vi "CD Init.vi"(8 "Error (in)":errorcluster, 11 "Device Reference":T10 format="%.0x") -> (0 "Error (out)":errorcluster, 1 "Inline Status Channels Refs":T3[](array[typedef]) format="%.0x", 2 "Card Parameters (out)":T22, 3 "RT Inline Data_Data Description_Channels":T13[](array[typedef]) {"Broadcast Frame Descriptors"."RTs"."Status Channel Ref" format="%.0x"; "Broadcast Frame Descriptors"."RTs"."Timestamp Channel Data Reference" format="%.0x"; "Broadcast Frame Descriptors"."BC"."Status Channel Refs" format="%.0x"; "Broadcast Frame Descriptors"."BC"."Words Block Data Refs"."Data Reference" format="%.0x"; "Broadcast Frame Descriptors"."BC"."Timestamp Channel Data Reference" format="%.0x"; "Frame Drescriptors"."RT"."Status Channel Ref" format="%.0x"; "Frame Drescriptors"."RT"."Words Block Data Refs"."Data Reference" format="%.0x"; "Frame Drescriptors"."RT"."Timestamp Channel Data Reference" format="%.0x"; "Frame Drescriptors"."BC"."Status Channel Refs" format="%.0x"; "Frame Drescriptors"."BC"."Words Block Data Refs"."Data Reference" format="%.0x"; "Frame Drescriptors"."BC"."Timestamp Channel Data Reference" format="%.0x"}, 6 "RT Async Data":T1 {"Map (MC Tx)"."Word Data Reference" format="%.0x"; "Map (MC Rx)"."Channel Data Reference" format="%.0x"; "Map (RT Command Channels)"."RT Command Channel Ref" format="%.0x"; "MAP (BC Acyclic Messages Trigger)"."Acyclic Message Trigger Channel Ref" format="%.0x"; "Map (Bc Command Channels)"."BC Command Channel Ref" format="%.0x"; "Map (RT to ..)"."Word Data Reference" format="%.0x"; "Map (BC to RT)"."Channel Data Reference" format="%.0x"})   [LabVIEW 2017, in "Ballard MIL-1553 Engine.lvlib"]
doc: "This VI reads all properties, creates different Maps (Tx) and initializes the Core of the board using XML file. Initialization is done here because Rx part is done Inline and Tx part asynchronously."
uses:
  Ballard MIL-1553 Engine.lvlib
  <vilib>/NI Veristand/Custom Device API/Custom Device Item Ref.ctl
  Controls/Card Parameters.ctl
  Shared/Controls and Global/Initialization Method.ctl
  Controls/RT Inline Data_Data Description_Channel.ctl
  Controls/RT Inline Frame Descriptor.ctl
  Controls/RT Inline Frame Descriptor_BC.ctl
  <vilib>/NI Veristand/Custom Device API/Data Reference.ctl
  <vilib>/NI Veristand/Custom Device API/Block Data Reference.ctl
  Controls/RT Inline Frame Descriptor_RT.ctl
  Shared/Controls and Global/RT CWD2.ctl
  Shared/Controls and Global/RT CWD1.ctl
  Shared/Controls and Global/RT messageType.ctl
  Controls/RT Inline Broadcast Frame Descriptor.ctl
  Controls/RT Async Data.ctl
  Controls/RT Async_Map BC2RT.ctl
  Controls/RT Async_Map_Type.ctl
  Controls/RT Async_Raw Values.ctl
  Controls/RT Async_Raw Values to Messages Index_Association.ctl
  Controls/RT Async_Map RT2BC.ctl
  Controls/RT Async_Map RTs Status.ctl
  Controls/RT Async_Map BC Command Channels.ctl
  Controls/RT Async_Map BC Acyclic Messages Trigger.ctl
  Controls/RT Async_Map RT Command Channels.ctl
  Controls/RT Init States.ctl
  Shared/Controls and Global/Compiled.Settings.ctl
  Shared/Controls and Global/RT Channel.ctl
  Shared/Controls and Global/RT BC.ctl
  Shared/Controls and Global/RT Message.ctl
  Shared/Controls and Global/RT Remote Terminal.ctl
  Shared/Controls and Global/RT Remote Terminal_rtMode.ctl
  Shared/Controls and Global/RT Remote Terminal_RT subAddress.ctl
  Shared/Controls and Global/RT Remote Terminal_RT direction.ctl
  Shared/Controls and Global/RT Remote Terminal_RT Mode Code.ctl
  Shared/Controls and Global/Global.vi
  <vilib>/NI Veristand/Custom Device API/Get Item Property (I32).vi
  <vilib>/NI Veristand/Custom Device API/Get Item Property (U16).vi
  <vilib>/NI Veristand/Custom Device API/Get Item Property (Variant).vi
  <vilib>/NI VeriStand/Custom Device API/Custom Device API.lvlib
  <vilib>/NI VeriStand/Custom Device Tools/Custom Device Utility Library/Custom Device Utility Library.lvlib
  Shared/Ballard 1553 Shared.lvlib
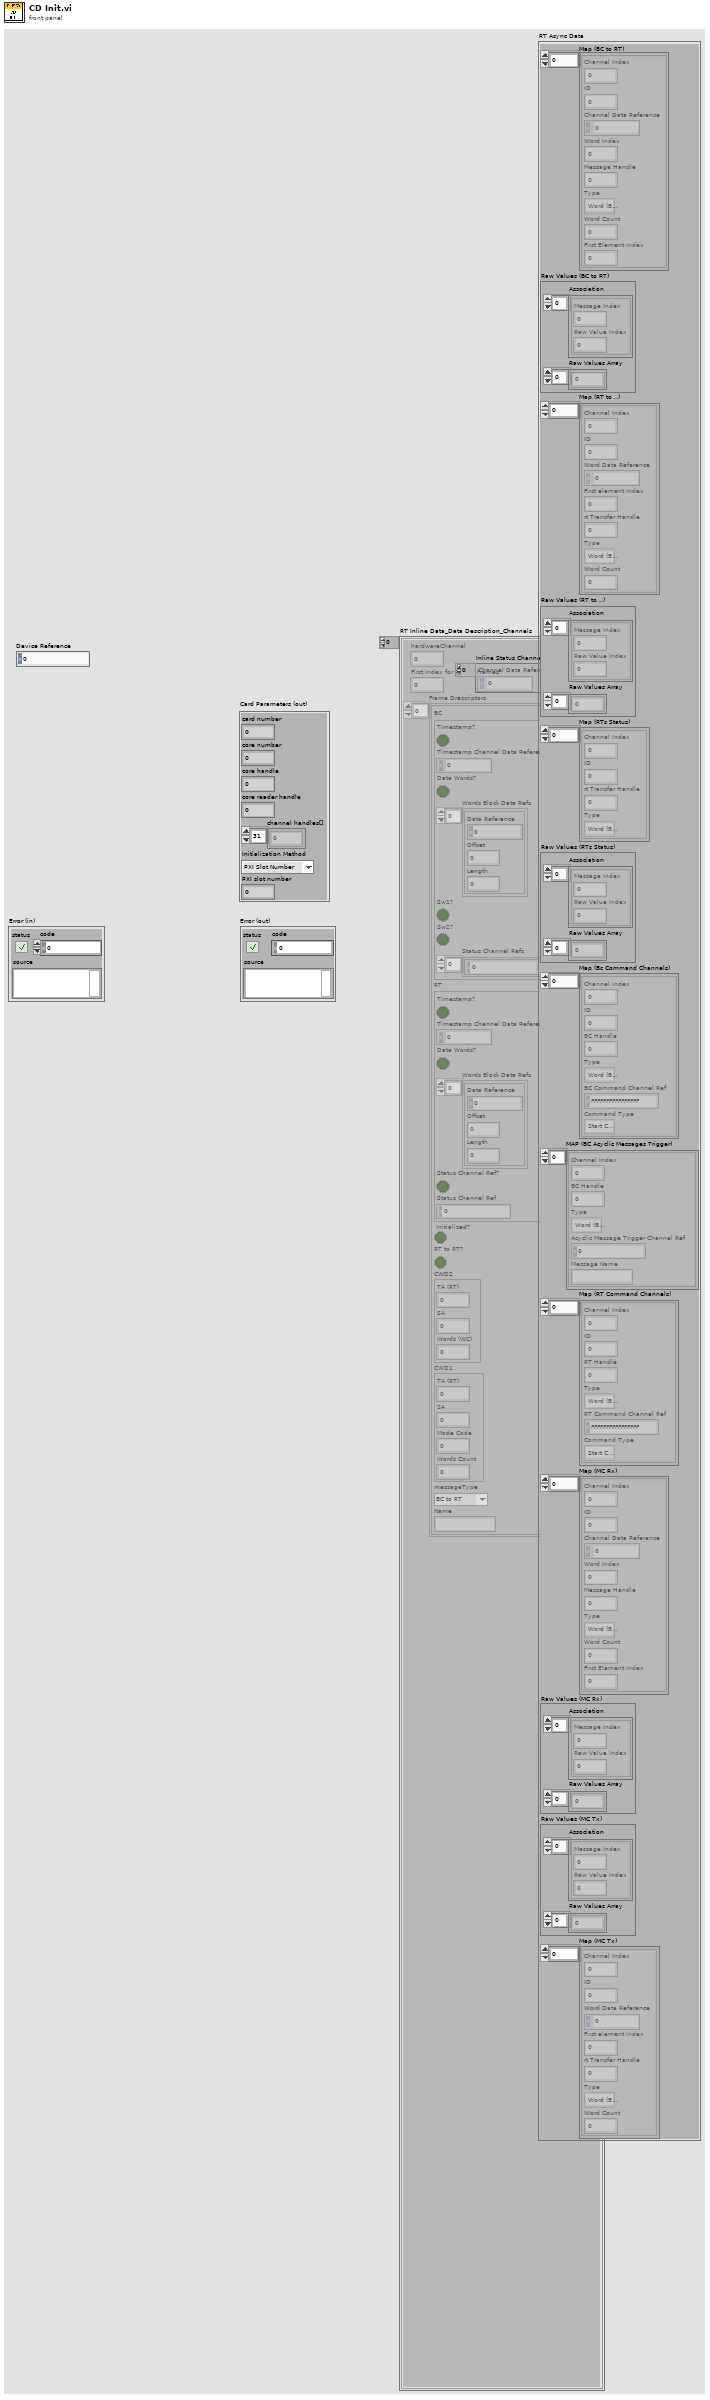
[diagram p1: front panel]
types:
  T1 = typedef "Ballard MIL-1553 Engine.lvlib/RT Async Data.ctl" = cluster{"Map (BC to RT)":T2[], "Raw Values (BC to RT)":T5, "Map (RT to ..)":T7[], "Raw Values (RT to ..)":T5, "Map (RTs Status)":T8[], "Raw Values (RTs Status)":T5, "Map (Bc Command Channels)":T9[], "MAP (BC Acyclic Messages Trigger)":T11[], "Map (RT Command Channels)":T12[], "Map (MC Rx)":T2[], "Raw Values (MC Rx)":T5, "Raw Values (MC Tx)":T5, "Map (MC Tx)":T7[]}
  T2 = typedef "Ballard MIL-1553 Engine.lvlib/RT Async_Map BC2RT.ctl" = cluster{"Channel Index":i32, "ID":i32, "Channel Data Reference":T3, "Word Index":i32, "Message Handle":u64, "Type":T4, "Word Count":i32, "First Element Index":i32}
  T3 = typedef "Custom Device API.lvlib/Data Reference.ctl" = i32
  T4 = typedef "Ballard MIL-1553 Engine.lvlib/RT Async_Map_Type.ctl" = enum16{"Word (BC to RT)", "Word (MC (Rx))", "Acyclic Message Trigger", "Word (RT to ..)", "Word (RT to RT)", "Word (MC (Tx))", "RT Status", "BC Commands", "RT Commands"}
  T5 = typedef "Ballard MIL-1553 Engine.lvlib/RT Async_Raw Values.ctl" = cluster{"Association":T6[], "Raw Values Array":u16[]}
  T6 = typedef "Ballard MIL-1553 Engine.lvlib/RT Async_Raw Values to Messages Index_Association.ctl" = cluster{"Message Index":i32, "Raw Value Index":i32}
  T7 = typedef "Ballard MIL-1553 Engine.lvlib/RT Async_Map RT2BC.ctl" = cluster{"Channel Index":i32, "ID":i32, "Word Data Reference":T3, "First element Index":i32, "rt Transfer Handle":u64, "Type":T4, "Word Count":i32}
  T8 = typedef "Ballard MIL-1553 Engine.lvlib/RT Async_Map RTs Status.ctl" = cluster{"Channel Index":i32, "ID":i32, "rt Transfer Handle":u64, "Type":T4}
  T9 = typedef "Ballard MIL-1553 Engine.lvlib/RT Async_Map BC Command Channels.ctl" = cluster{"Channel Index":i32, "ID":i32, "BC Handle":u64, "Type":T4, "BC Command Channel Ref":T10, "Command Type":enum16{"Start Command", "Stop Command"}}
  T10 = typedef "Custom Device API.lvlib/Custom Device Item Ref.ctl" = u64
  T11 = typedef "Ballard MIL-1553 Engine.lvlib/RT Async_Map BC Acyclic Messages Trigger.ctl" = cluster{"Channel Index":i32, "BC Handle":u64, "Type":T4, "Acyclic Message Trigger Channel Ref":T10, "Message Name":string}
  T12 = typedef "Ballard MIL-1553 Engine.lvlib/RT Async_Map RT Command Channels.ctl" = cluster{"Channel Index":i32, "ID":i32, "RT Handle":u64, "Type":T4, "RT Command Channel Ref":T10, "Command Type":enum16{"Start Command", "Stop Command"}}
  T13 = typedef "Ballard MIL-1553 Engine.lvlib/RT Inline Data_Data Description_Channel.ctl" = cluster{"hardwareChannel":u16, "First Index for RT2RT Frames":i32, "Frame Drescriptors":T14[], "Broadcast Frame Descriptors":T21[]}
  T14 = typedef "Ballard MIL-1553 Engine.lvlib/RT Inline Frame Descriptor.ctl" = cluster{"BC":T15, "RT":T17, "Initialized?":bool, "RT to RT?":bool, "CWD2":T18, "CWD1":T19, "messageType":T20, "Name":string}
  T15 = typedef "Ballard MIL-1553 Engine.lvlib/RT Inline Frame Descriptor_BC.ctl" = cluster{"Timestamp?":bool, "Timestamp Channel Data Reference":T3, "Data Words?":bool, "Words Block Data Refs":T16[], "Sw1?":bool, "Sw2?":bool, "Status Channel Refs":T10[]}
  T16 = typedef "Custom Device API.lvlib/Block Data Reference.ctl" = cluster{"Data Reference":T3, "Offset":u64, "Length":u64}
  T17 = typedef "Ballard MIL-1553 Engine.lvlib/RT Inline Frame Descriptor_RT.ctl" = cluster{"Timestamp?":bool, "Timestamp Channel Data Reference":T3, "Data Words?":bool, "Words Block Data Refs":T16[], "Status Channel Ref?":bool, "Status Channel Ref":T10}
  T18 = typedef "Ballard 1553 Shared.lvlib/RT CWD2.ctl" = cluster{"TA (RT)":i8, "SA":i8, "Words (WC)":i8}
  T19 = typedef "Ballard 1553 Shared.lvlib/RT CWD1.ctl" = cluster{"TA (RT)":i8, "SA":i8, "Mode Code":i8, "Words Count":i8}
  T20 = typedef "Ballard 1553 Shared.lvlib/RT messageType.ctl" = enum16{"BC to RT", "RT to BC", "RT to RT", "MC (Rx)", "MC (Tx)"}
  T21 = typedef "Ballard MIL-1553 Engine.lvlib/RT Inline Broadcast Frame Descriptor.ctl" = cluster{"BC":T15, "Initialized?":bool, "RT to RT?":bool, "CWD2":T18, "CWD1":T19, "messageType":T20, "Name":string, "RTs":T17[]}
  T22 = typedef "Ballard MIL-1553 Engine.lvlib/Card Parameters.ctl" = cluster{"card number":i32, "core number":i32, "core handle":u64, "core reader handle":u64, "channel handles[]":u64[], "Initialization Method":T23, "PXI slot number":i32}
  T23 = typedef "Ballard 1553 Shared.lvlib/Initialization Method.ctl" = enum16{"PXI Slot Number", "Card Number"}
  T24 = typedef "Ballard MIL-1553 Engine.lvlib/RT Init States.ctl" = enum16{"Initialization", "Get Card Settings", "Get Channel Count", "Parse Channels", "Ballard-1553 Initialize", "Get Status Channels Reference", "Exit"}
  T25 = typedef "Ballard 1553 Shared.lvlib/Compiled.Settings.ctl" = cluster{"Name":string, "channels":T26[]}
  T26 = typedef "Ballard 1553 Shared.lvlib/RT Channel.ctl" = cluster{"name":string, "hardWare Channel Number":u16, "BC":T27, "RTs":T29[]}
  T27 = typedef "Ballard 1553 Shared.lvlib/RT BC.ctl" = cluster{"ID":i32, "name":string, "Command Channels Refs":T10[], "messages":T28[], "Acyclic Frames Trigger Channels Refs":T10[], "Acyclic Frames Names":string[]}
  T28 = typedef "Ballard 1553 Shared.lvlib/RT Message.ctl" = cluster{"Name":string, "messageType":T20, "CWD1":T19, "CWD2":T18, "Status Channel Data Refs":T3[], "Words Item Refs":T10[], "Words Block Data Refs":T16[], "Words Values Array":u16[], "Timestamp Channel Data Reference":T3, "ID":i32, "Timestamp?":bool, "Data Words?":bool, "Status Channel Ref?":bool}
  T29 = typedef "Ballard 1553 Shared.lvlib/RT Remote Terminal.ctl" = cluster{"ID":i32, "name":string, "RT Address":i32, "rtMode":T30, "Command Channels Refs":T10[], "Status Channel Data Reference":T3, "subAddresses":T31[], "Mode Codes":T33[]}
  T30 = typedef "Ballard 1553 Shared.lvlib/RT Remote Terminal_rtMode.ctl" = enum16{"Simulate", "Monitor", "Disable"}
  T31 = typedef "Ballard 1553 Shared.lvlib/RT Remote Terminal_RT subAddress.ctl" = cluster{"name":string, "subAddress":i8, "direction":T32, "Timestamp Channel Data Reference":T3, "Words Values Array":u16[], "Words Block Data Refs":T16[], "Words Item Refs":T10[], "ID":i32, "Timestamp?":bool, "Data Words?":bool}
  T32 = typedef "Ballard 1553 Shared.lvlib/RT Remote Terminal_RT direction.ctl" = enum16{"Tx", "Rx"}
  T33 = typedef "Ballard 1553 Shared.lvlib/RT Remote Terminal_RT Mode Code.ctl" = cluster{"name":string, "direction":T32, "Timestamp Channel Data Reference":T3, "Words Values Array":u16[], "Words Block Data Refs":T16[], "Words Item Refs":T10[], "ID":i32, "Timestamp?":bool, "Data Words?":bool, "Code Number":i32}
  T34 = typedef "Custom Device API.lvlib/Custom Device File Dependency.ctl" = cluster{"Source":T35, "RT Destination":path, "ForceDownload?":bool, "SupportedTarget":T37, "Version":string}
  T35 = typedef "Custom Device API.lvlib/Path Specification.ctl" = cluster{"Path":path, "Type":T36}
  T36 = typedef "Custom Device API.lvlib/Path Type.ctl" = enum16{"Absolute", "To Base", "To Common Data Dir", "To Application Data Dir"}
  T37 = typedef "Custom Device API.lvlib/Custom Device Supported Target.ctl" = enum16{"All", "PharLap", "VxWorks", "Windows", "Linux_32_ARM", "Linux_x64", "PharLap & Windows", "PharLap & VxWorks", "VxWorks & Windows"}
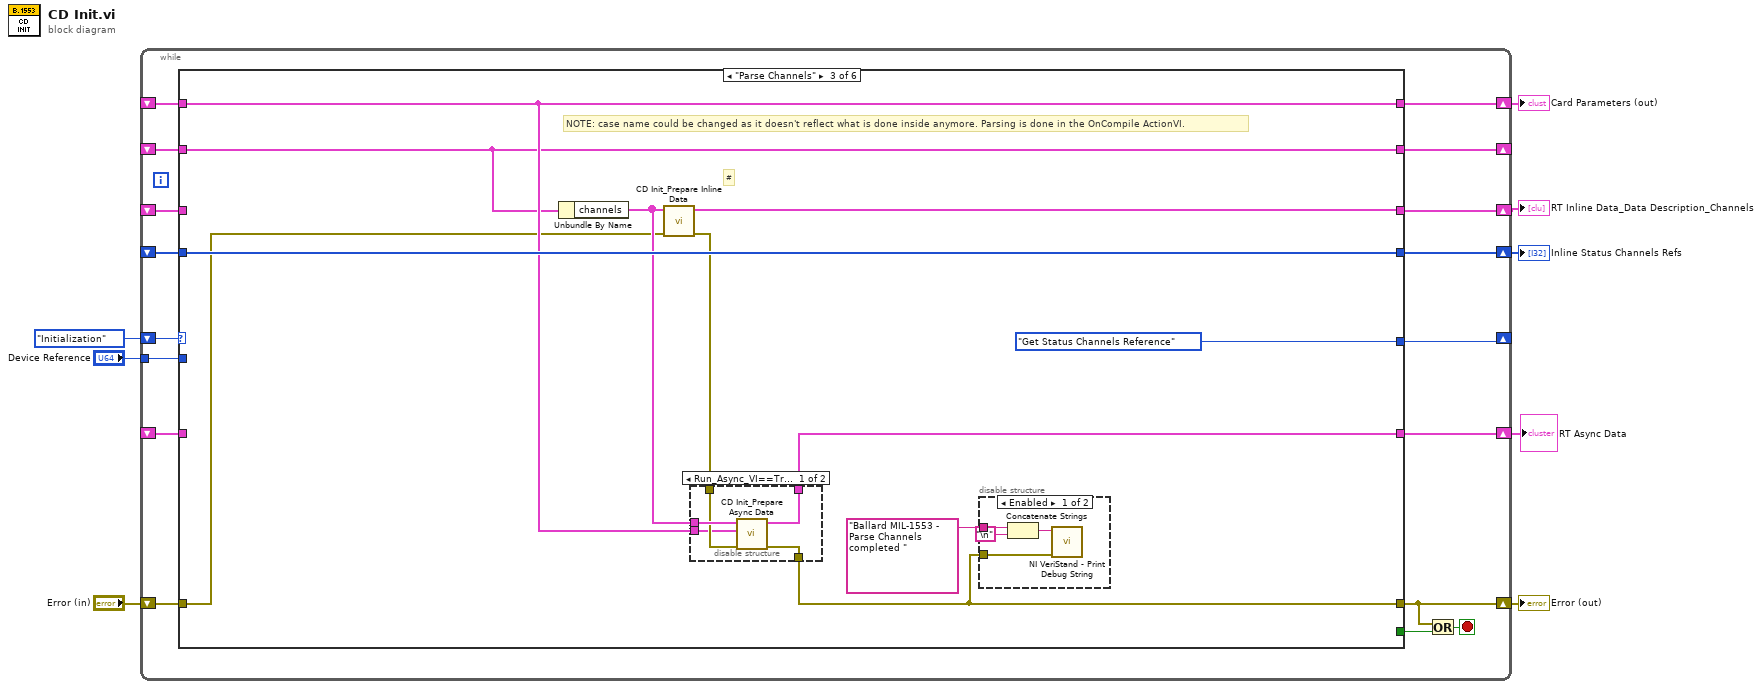
[diagram p0: block diagram]
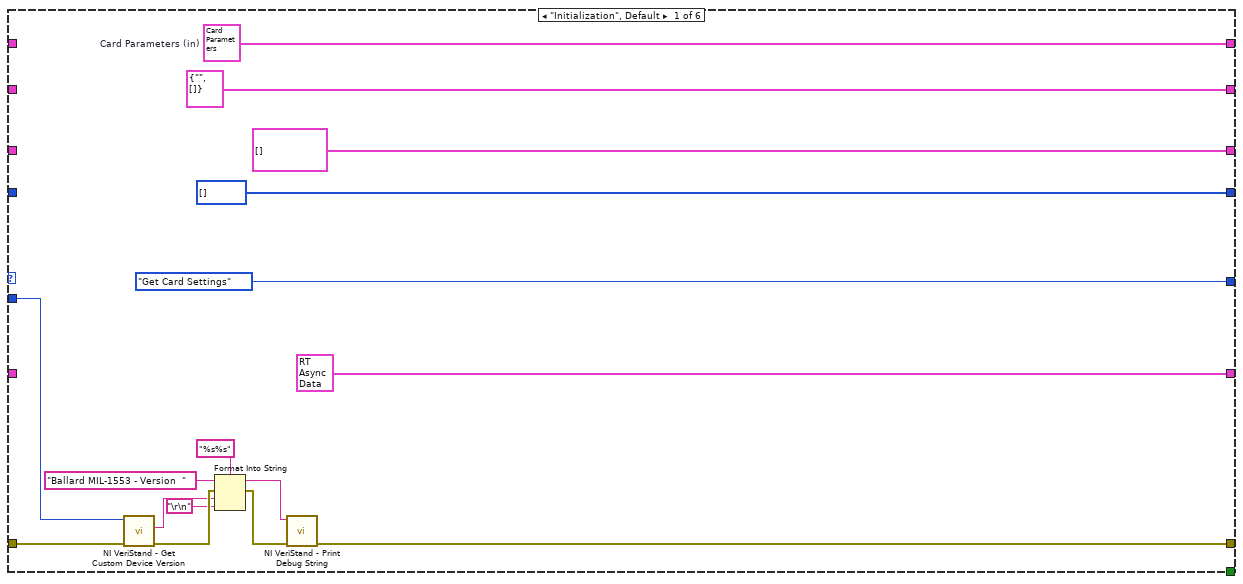
[diagram p2: hidden frame]
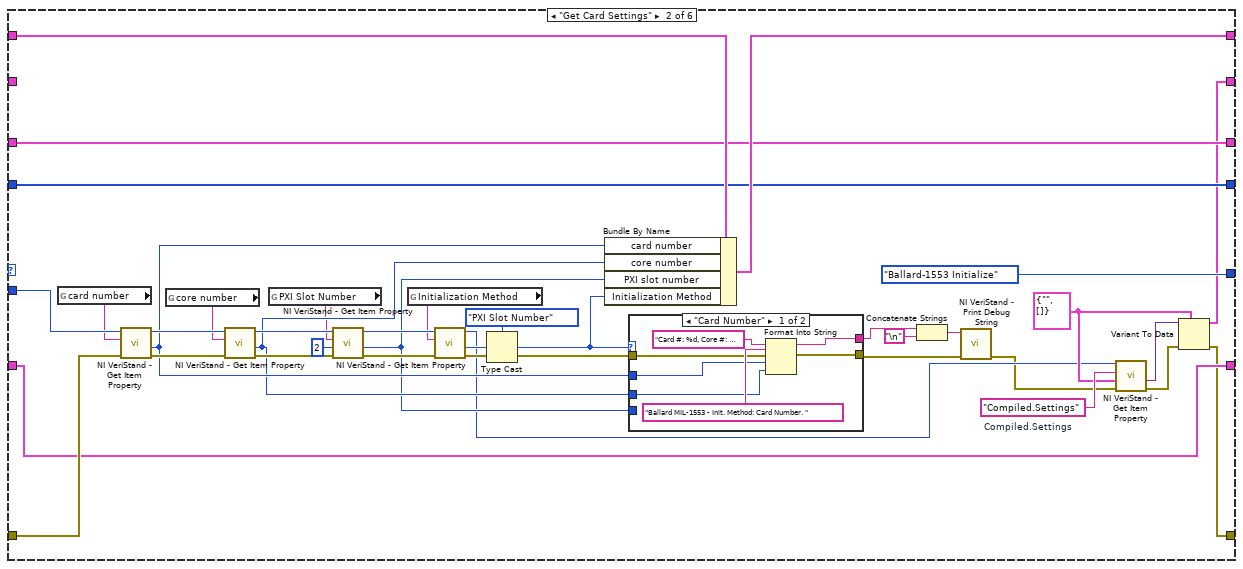
[diagram p3: hidden frame]
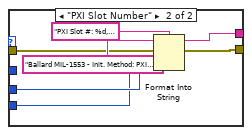
[diagram p4: hidden frame]
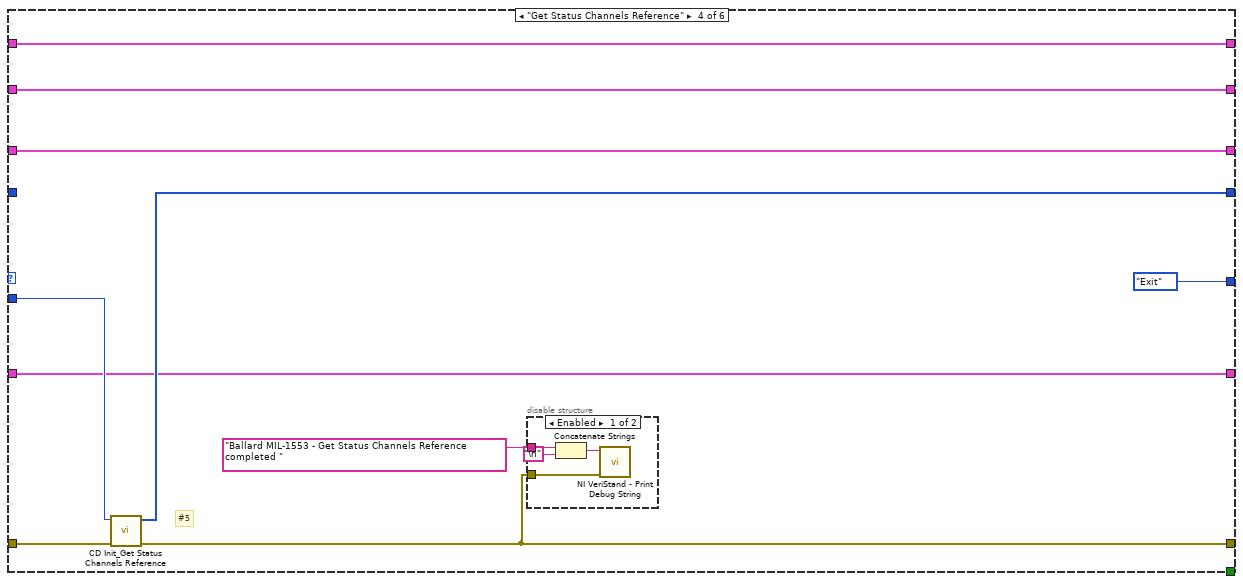
[diagram p7: hidden frame]
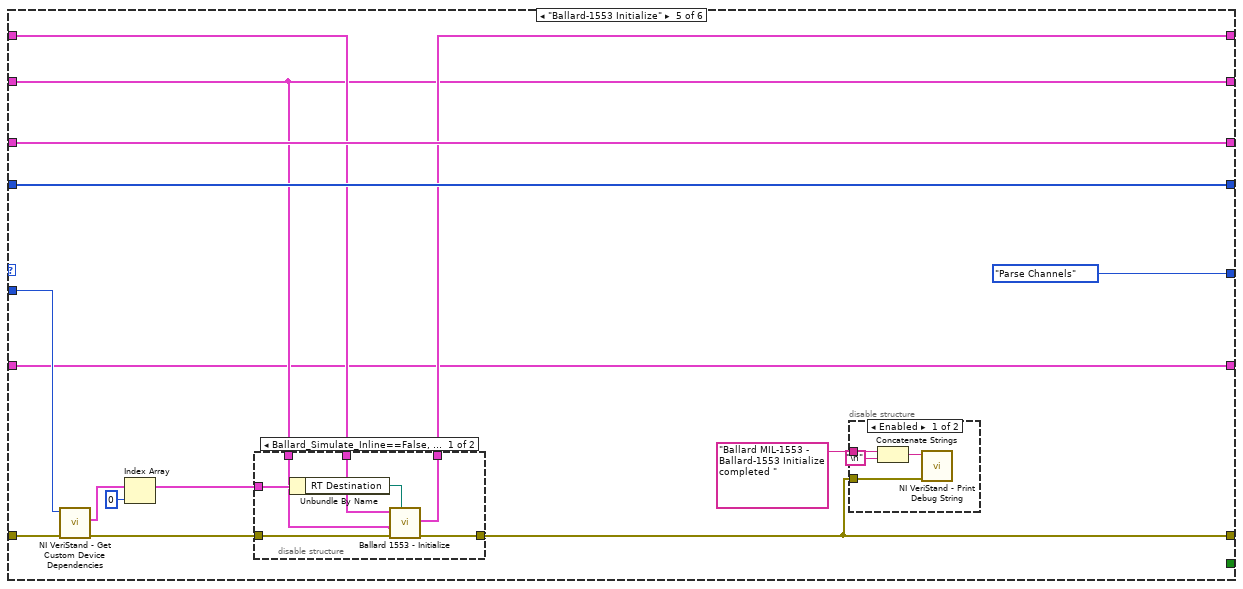
[diagram p9: hidden frame]
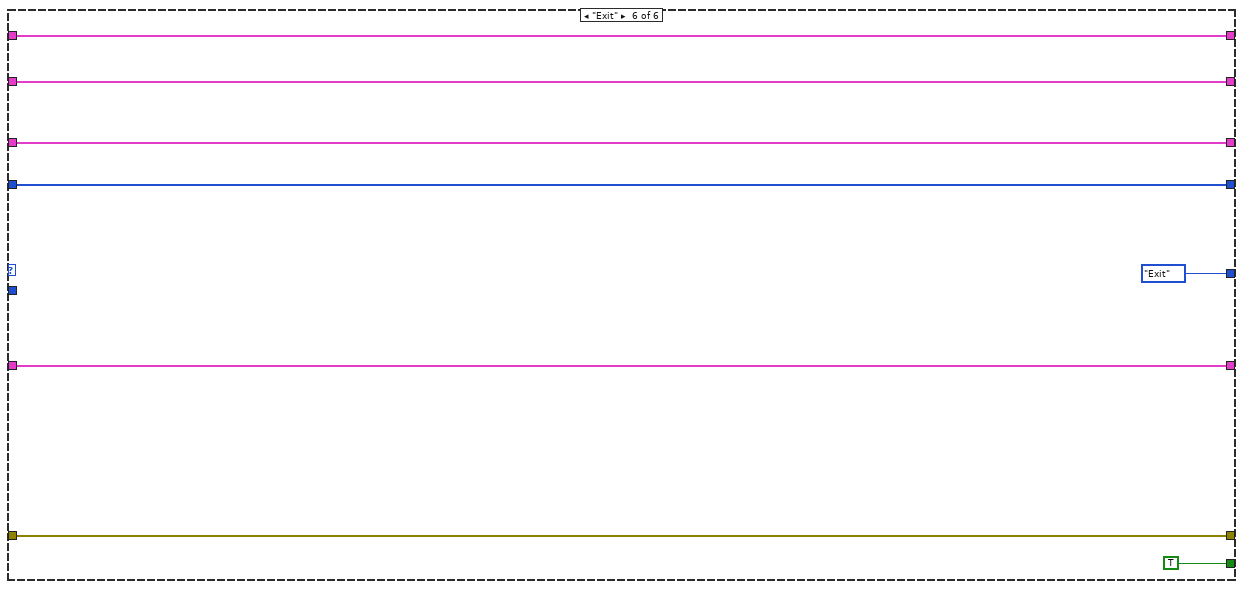
[diagram p12: hidden frame]
diagram:
  n1 = while {
    shift-right: [w24] -> _
    shift-left: RT_Init_States."Initialization" -> [w18]
    tunnel: "Device Reference" -> [w23]
    shift-right: [w19] -> w4
    shift-left: _ -> [w20]
    shift-right: [w17] -> w2
    shift-left: _ -> [w16]
    shift-right: [w15] -> w3
    shift-left: _ -> [w14]
    shift-right: [w13] -> w6
    shift-left: "Error (in)" -> [w25]
    shift-right: [w12] -> _
    shift-left: _ -> [w11]
    shift-right: [w10] -> w1
    shift-left: _ -> [w9]
    stop <- w22 stop-if-true
    n2 = case shown="\"Parse Channels\"" w18 {
      tunnel: w25 -> [w38 w78 w96 w120 w140 w164]
      tunnel: [w36 w43 w94 w115 w129 w164] -> w13
      tunnel: [RT_Init_States."Get Card Settings" RT_Init_States."Ballard-1553 Initialize" RT_Init_States."Get Status Channels Reference" RT_Init_States."Exit" RT_Init_States."Parse Channels" RT_Init_States."Exit"] -> w24
      tunnel: w23 -> [w37 w75 _ w119 w139 _]
      tunnel: [_ _ _ _ _ TRUE] -> w21
      tunnel: w20 -> [_ w74 w100 w121 w133 w161]
      tunnel: [w40 w73 w100 w121 w136 w161] -> w19
      tunnel: [T13[] [] ("RT Inline Data_Data Description_Channels") w72 w102 w124 w138 w160] -> w17
      tunnel: w16 -> [_ w72 _ w124 w138 w160]
      tunnel: [i32[] [] w71 w103 w122 w137 w159] -> w15
      tunnel: w14 -> [_ w71 w103 _ w137 w159]
      tunnel: [T25 {"Name"="", "channels"=[]} ("Compiled.Settings") w42 w97 w118 w132 w158] -> w12
      tunnel: w11 -> [_ _ w97 w118 w132 w158]
      tunnel: [T1 {"Map (BC to RT)"=[], "Raw Values (BC to RT)"={"Association"=[], "Raw Values Array"=[]}, "Map (RT to ..)"=[], "Raw Values (RT to ..)"={"Association"=[], "Raw Values Array"=[]}, "Map (RTs Status)"=[], "Raw Values (RTs Status)"={"Association"=[], "Raw Values Array"=[]}, "Map (Bc Command Channels)"=[], "MAP (BC Acyclic Messages Trigger)"=[], "Map (RT Command Channels)"=[], "Map (MC Rx)"=[], "Raw Values (MC Rx)"={"Association"=[], "Raw Values Array"=[]}, "Raw Values (MC Tx)"={"Association"=[], "Raw Values Array"=[]}, "Map (MC Tx)"=[]} ("RT Async Data") w50 w99 w117 w131 w157] -> w10
      tunnel: w9 -> [_ w50 _ w117 w131 w157]
      frame "Initialization", Default {
        w40 = T22 {"card number"=0, "core number"=0, "core handle"=0, "core reader handle"=0, "channel handles[]"=[], "Initialization Method"=enum."PXI Slot Number", "PXI slot number"=0}  # Card Parameters (in)
        n3 = call <vilib>:"NI VeriStand - Get Custom Device Version.vi"("error in (no error)"=w38, "Device Ref in"=w37) -> ("error out"=w35:errorcluster, "Value"=w32:string)  [unwired: 7 in, 1 out]
        n4 = Format Into String(format string="%s%s", initial string="Ballard MIL-1553 - Version  ", error in=w35, w32, "\r\n") -> (resulting string=w30:string, error out=w34:errorcluster)
        n5 = call <vilib>:"NI VeriStand - Print Debug String.vi"("error in (no error)"=w34, "Message"=w30) -> ("error out"=w36:errorcluster)  [unwired: 9 in]
      }
      frame "Get Card Settings" {
        w47 = "Compiled.Settings"  # Compiled.Settings
        w46 = T25 {"Name"="", "channels"=[]} ("Compiled.Settings")
        n6 = global read "Global.vi" "card number"() -> (w51:string)
        n7 = call-poly <vilib>:"NI VeriStand - Get Item Property.vi"("error in (no error)"=w78, "Property Name"=w51, "Item Ref in"=w75) -> ("error out"=w77:errorcluster, "Value"=w59:i32, "Item Ref out"=w79:T10)  [unwired: 5 in, 1 out]
        n8 = global read "Global.vi" "core number"() -> (w52:string)
        n9 = call-poly <vilib>:"NI VeriStand - Get Item Property.vi"("error in (no error)"=w77, "Property Name"=w52, "Item Ref in"=w79) -> ("error out"=w69:errorcluster, "Value"=w58:i32, "Item Ref out"=w70:T10)  [unwired: 5 in, 1 out]
        n10 = global read "Global.vi" "PXI Slot Number"() -> (w53:string)
        n11 = call-poly <vilib>:"NI VeriStand - Get Item Property.vi"("error in (no error)"=w69, "Default Value"=2, "Property Name"=w53, "Item Ref in"=w70) -> ("error out"=w67:errorcluster, "Value"=w57:i32, "Item Ref out"=w66:T10)  [unwired: 4 in, 1 out]
        n12 = global read "Global.vi" "Initialization Method"() -> (w54:string)
        n13 = call-poly <vilib>:"NI VeriStand - Get Item Property.vi"("error in (no error)"=w67, "Property Name"=w54, "Item Ref in"=w66) -> ("error out"=w56:errorcluster, "Value"=w65:u16, "Item Ref out"=w45:T10)  [unwired: 5 in, 1 out]
        n14 = Type Cast(type=Initialization_Method."PXI Slot Number" ("Initialization Method"), x=w65) -> (*(type *) &x=w63:T23)
        n15 = Bundle By Name(cluster=w74, "card number"=w59, "core number"=w58, "PXI slot number"=w57, "Initialization Method"=w63) -> (w73:T22)
        n16 = case shown="\"Card Number\"" w63 {
          tunnel: [w86 w93] -> w60
          tunnel: w59 -> [w83 _]
          tunnel: w58 -> [w82 w90]
          tunnel: w57 -> [_ w89]
          tunnel: w56 -> [w81 w88]
          tunnel: [w80 w87] -> w55
          frame "Card Number" {
            n17 = Format Into String(format string="Card #: %d, Core #: %d.", initial string="Ballard MIL-1553 - Init. Method: Card Number. " ("String to write"), error in=w81, w83, w82) -> (resulting string=w86:string, error out=w80:errorcluster)
          }
          frame "PXI Slot Number" {
            n18 = Format Into String(format string="PXI Slot #: %d, Core #: %d.", initial string="Ballard MIL-1553 - Init. Method: PXI Slot Number. " ("String to write"), error in=w88, w89, w90) -> (resulting string=w93:string, error out=w87:errorcluster)
          }
        }
        n19 = Concatenate Strings(w60, "\n") -> (w62:string)
        n20 = call <vilib>:"NI VeriStand - Print Debug String.vi"("error in (no error)"=w55, "Message"=w62) -> ("error out"=w44:errorcluster)  [unwired: 9 in]
        n21 = call-poly <vilib>:"NI VeriStand - Get Item Property.vi"("error in (no error)"=w44, "Default Value"=w46, "Property Name"=w47, "Item Ref in"=w45) -> ("error out"=w49:errorcluster, "Value"=w48:variant)  [unwired: 4 in, 2 out]
        n22 = Variant To Data(error in=w49, type=w46, Variant=w48) -> (data=w42:T25, error out=w43:errorcluster)
      }
      frame "Parse Channels" {
        # "#"
        # "NOTE: case name could be changed as it doesn't reflect what is done inside anymore. Parsing is done in the OnCompile ActionVI."
        n23 = Unbundle By Name(w97) -> ("channels"=w101:T26[])
        n24 = call "CD Init_Prepare Inline Data.vi"("error in (no error)"=w96, "channels In"=w101) -> ("error out"=w95:errorcluster, "RT Inline Data_Data Description_Channels"=w102:T13[])  [unwired: 8 in]
        n25 = disable-structure shown="Run_Async_VI==True, Default" {
          disable-tunnel: w101 -> [w109 _]
          disable-tunnel: w95 -> [w108 w110]
          disable-tunnel: w100 -> [w107 _]
          disable-tunnel: [w106 _] -> w99
          disable-tunnel: [w105 w110] -> w94
          frame condition #0 (active) {
            n26 = call "CD Init_Prepare Async Data.vi"("error in (no error)"=w108, "Card Parameters (in)"=w107, "Channels In"=w109) -> ("error out"=w105:errorcluster, "RT Async Data"=w106:T1)  [unwired: 7 in]
          }
          frame condition #1 {
          }
        }
        n27 = disable-structure shown="Enabled" {
          disable-tunnel: w94 -> [w112 _]
          disable-tunnel: "Ballard MIL-1553 - Parse Channels completed " -> [w111 _]
          frame Enabled {
            n28 = Concatenate Strings(w111, "\n") -> (w113:string)
            n29 = call <vilib>:"NI VeriStand - Print Debug String.vi"("error in (no error)"=w112, "Message"=w113) -> ()  [unwired: 9 in, 1 out]
          }
          frame Disabled {
          }
        }
      }
      frame "Get Status Channels Reference" {
        # "#5"
        n30 = call "CD Init_Get Status Channels Reference.vi"("error in (no error)"=w120, "Device Reference"=w119) -> ("error out"=w115:errorcluster, "Array"=w122:T3[])  [unwired: 8 in]
        n31 = disable-structure shown="Enabled" {
          disable-tunnel: w115 -> [w126 _]
          disable-tunnel: "Ballard MIL-1553 - Get Status Channels Reference completed " -> [w125 _]
          frame Enabled {
            n32 = Concatenate Strings(w125, "\n") -> (w127:string)
            n33 = call <vilib>:"NI VeriStand - Print Debug String.vi"("error in (no error)"=w126, "Message"=w127) -> ()  [unwired: 9 in, 1 out]
          }
          frame Disabled {
          }
        }
      }
      frame "Ballard-1553 Initialize" {
        n34 = call <vilib>:"NI VeriStand - Get Custom Device Dependencies.vi"("error in (no error)"=w140, "Device Ref in"=w139) -> ("error out"=w134:errorcluster, "Dependencies"=w142:T34[])  [unwired: 7 in, 1 out]
        n35 = Index Array(array=w142, index=0) -> (element=w141:T34)
        n36 = disable-structure shown="Ballard_Simulate_Inline==False, Default" {
          disable-tunnel: w141 -> [w150 _]
          disable-tunnel: [w148 w151] -> w136
          disable-tunnel: w134 -> [w147 w152]
          disable-tunnel: w133 -> [w146 w151]
          disable-tunnel: w132 -> [w145 _]
          disable-tunnel: [w144 w152] -> w129
          frame condition #0 (active) {
            n37 = Unbundle By Name(w150) -> ("RT Destination"=w149:path)
            n38 = call "Ballard 1553 - Initialize.vi"("RT Config Filepath"=w149, "Error (in)"=w147, "Compiled.Settings"=w145, "Card Parameters (in)"=w146) -> ("Error (out)"=w144:errorcluster, "Card Parameters (out)"=w148:T22)  [unwired: 6 in]
          }
          frame condition #1 {
          }
        }
        n39 = disable-structure shown="Enabled" {
          disable-tunnel: w129 -> [w154 _]
          disable-tunnel: "Ballard MIL-1553 - Ballard-1553 Initialize completed " -> [w153 _]
          frame Enabled {
            n40 = Concatenate Strings(w153, "\n") -> (w155:string)
            n41 = call <vilib>:"NI VeriStand - Print Debug String.vi"("error in (no error)"=w154, "Message"=w155) -> ()  [unwired: 9 in, 1 out]
          }
          frame Disabled {
          }
        }
      }
      frame "Exit" {
      }
    }
    n42 = Or(x=w13, y=w21) -> (x .or. y?=w22:bool)
  }
  "Error (out)" <- w6
  "Card Parameters (out)" <- w4
  "RT Inline Data_Data Description_Channels" <- w2
  "Inline Status Channels Refs" <- w3
  "RT Async Data" <- w1
